vi "addItem.vi"(8 "error in (no error)":errorcluster, 10 "Item.lvclass":refnum<class "Item.lvclass">, 11 "Meal in":refnum<class "Meal.lvclass">) -> (0 "error out":errorcluster, 3 "Meal out":refnum<class "Meal.lvclass">)   [LabVIEW 2017, in "Meal.lvclass"]
uses:
  Meal.lvclass
  Item Class/Item.lvclass
  Meal.lvclass/Meal.ctl
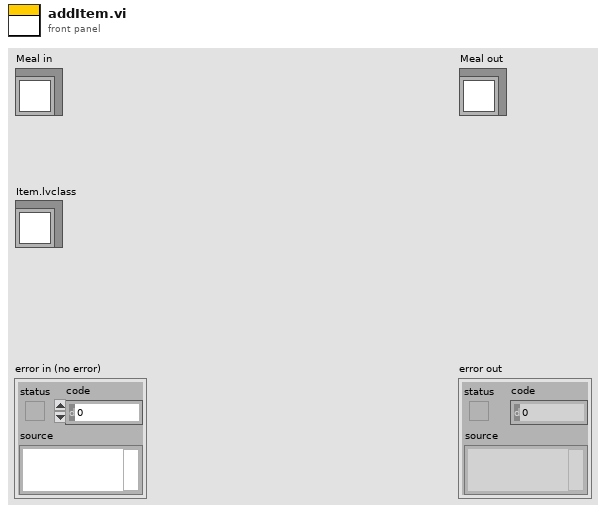
[diagram p1: front panel]
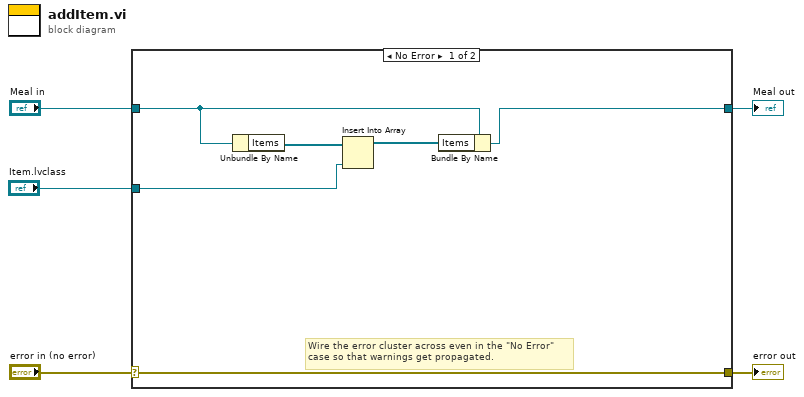
[diagram p0: block diagram]
diagram:
  n1 = case shown="No Error" "error in (no error)" {
    selector: "error in (no error)" -> [w11 w13]
    tunnel: [w11 w13] -> w4
    tunnel: [w9 w12] -> w2
    tunnel: "Meal in" -> [w10 w12]
    tunnel: "Item.lvclass" -> [w6 _]
    frame No Error {
      # "Wire the error cluster across even in the \"No Error\"\ncase so that warnings get propagated."
      n2 = Unbundle By Name(w10) -> ("Items"=w8:refnum<class "Item.lvclass">[])
      n3 = Insert Into Array(array=w8, new element=w6) -> (w7:refnum<class "Item.lvclass">[])  [unwired: 1 in]
      n4 = Bundle By Name(cluster=w10, "Items"=w7) -> (w9:refnum<class "Meal.lvclass">)
    }
    frame Error {
    }
  }
  "error out" <- w4
  "Meal out" <- w2
